vi "Charge_On_Magnet_Off.vi"() -> ()   [LabVIEW 2010]
uses:
  <vilib>/SwitchExecutive/nise.llb/niSE Multiconnect Mode Enum.ctl
  <instrlib>/Keithley 24XX/Keithley 24XX.lvlib
panel:
  in  "Apply Loads":bool
  out "Instruments Ready":bool
  in  "Release Instruments":bool
  in  "Initialize Instruments":bool
  in  "Apply Magnet":bool
  in  "Apply Charge":bool
  # "CHARGE"
  # "MAGNET"
  # "SETUP"
  # "LOADS"
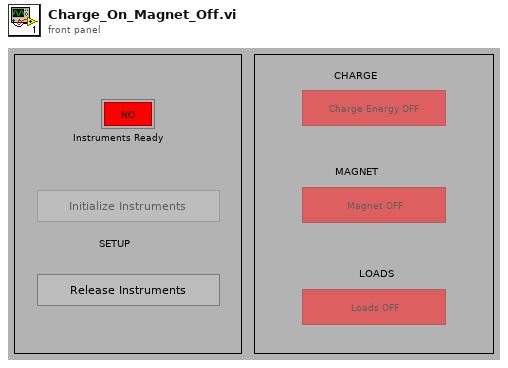
[diagram p1: front panel]
types:
  T1 = enum8{"Enabled", "Disabled", "Disabled and Grayed Out"}
  T2 = typedef "niSE Multiconnect Mode Enum.ctl" = i32
  T3 = typedef "niSE SessionRefnum.ctl" = refnum<k1>
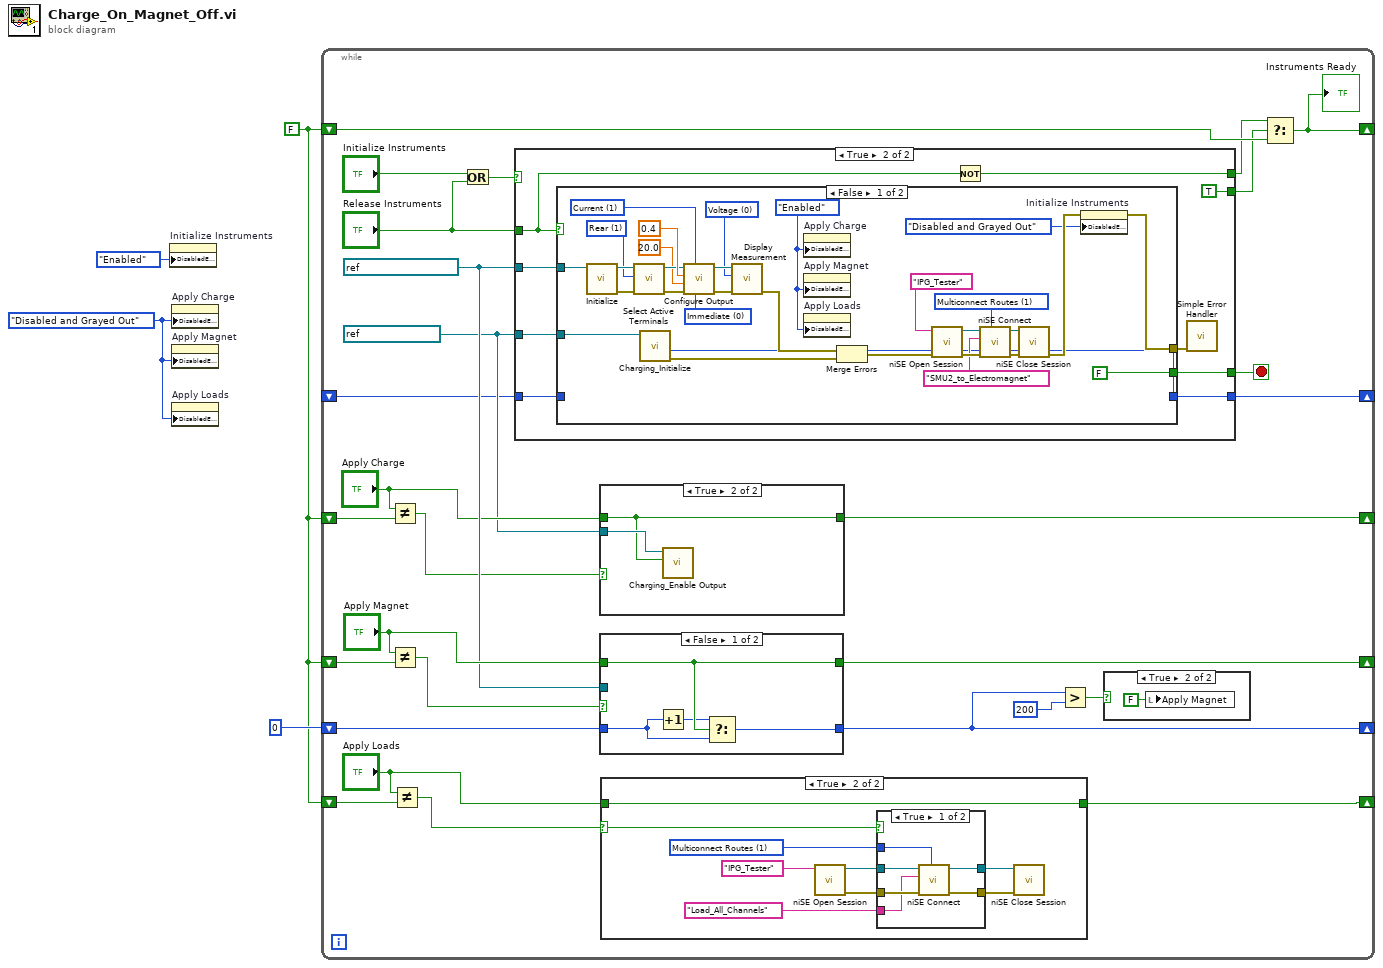
[diagram p0: block diagram]
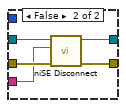
[diagram p3: hidden frame]
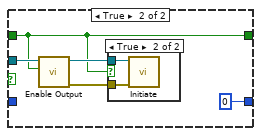
[diagram p6: hidden frame]
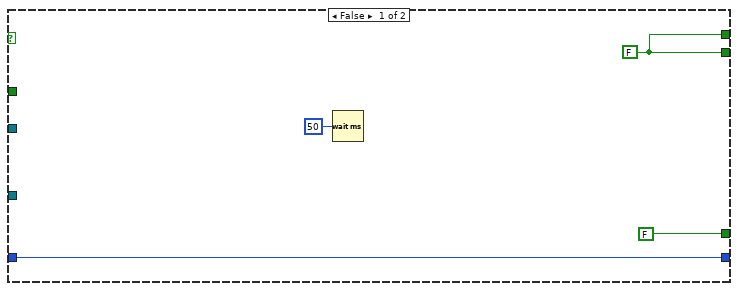
[diagram p8: hidden frame]
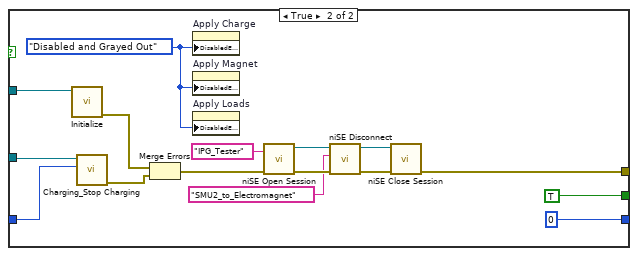
[diagram p9: hidden frame]
diagram:
  w1 = T1."Disabled and Grayed Out" ("Disabled")
  w2 = FALSE
  n1 = property on="Initialize Instruments" class="Bool"("DisabledEnum"=T1."Enabled" ("Disabled")) -> ()  [unwired: 2 in, 2 out]
  n2 = property on="Apply Charge" class="Bool (strict)"("DisabledEnum"=w1) -> ()  [unwired: 2 in, 2 out]
  n3 = property on="Apply Magnet" class="Bool (strict)"("DisabledEnum"=w1) -> ()  [unwired: 2 in, 2 out]
  n4 = property on="Apply Loads" class="Bool (strict)"("DisabledEnum"=w1) -> ()  [unwired: 2 in, 2 out]
  n5 = while {
    shift-right: [w32] -> _
    shift-left: w2 -> [w31]
    shift-right: [w13] -> _
    shift-left: w2 -> [w29]
    shift-right: [w19] -> _
    shift-left: w2 -> [w30]
    shift-right: [w17] -> _
    shift-left: u32 0 -> [w22]
    shift-right: [w8] -> _
    shift-left: w2 -> [w11]
    shift-right: [w6] -> _
    shift-left: _ -> [w5]
    stop <- w12 stop-if-true
    w7 = refnum<k15> "IVI-AG33210A" ("logical name (\"SampleFGen\")")
    w20 = refnum<visa-resource-name> "GPIB0::10::INSTR" ("VISA resource name")
    n6 = Not Equal?(x="Apply Charge", y=w29) -> (x != y?=w15:bool)
    n7 = Not Equal?(x="Apply Magnet", y=w30) -> (x != y?=w23:bool)
    n8 = Not Equal?(x="Apply Loads", y=w11) -> (x != y?=w10:bool)
    n9 = Or(x="Initialize Instruments", y="Release Instruments") -> (x .or. y?=w27:bool)
    n10 = case shown="True" w27 {
      tunnel: [w72 TRUE] -> w26
      tunnel: [w72 w80] -> w25
      tunnel: "Release Instruments" -> [_ w78]
      tunnel: w20 -> [_ w79]
      tunnel: w7 -> [_ w77]
      tunnel: [FALSE w75] -> w12
      tunnel: [w69 w74] -> w6
      tunnel: w5 -> [w69 w73]
      frame False {
        w72 = FALSE
        n11 = Wait (ms)(milliseconds to wait=u32 50) -> ()  [unwired: 1 out]
      }
      frame True {
        n12 = case shown="False" w78 {
          tunnel: w79 -> [w111 w127]
          tunnel: w77 -> [w82 w115]
          tunnel: [w87 w120] -> w76
          tunnel: [FALSE TRUE] -> w75
          tunnel: [w83 0 ("Arbitrary Waveform Handle [ARB]")] -> w74
          tunnel: w73 -> [_ w112]
          frame False {
            w91 = u16 0 items=["Immediate", "Triggered"] ("Output Type  (0: Immediate)")
            w92 = u16 0 items=["Voltage", "Current", "Resistance"] ("Displayed Measurement (0: Voltage)")
            w85 = T1."Enabled" ("Disabled")
            w101 = T2 1 items=["Use Default Mode"=-1, "Multiconnect Routes"=1, "No Multiconnect"=0] ("Multiconnect Mode (Use Default Mode)")
            w103 = u16 1 items=["Voltage", "Current"] ("Source Mode  (0: Voltage)")
            w108 = u16 1 items=["Front", "Rear"] ("Active Terminals (0: Front)")
            n13 = call <instrlib>:"Initialize.vi"("VISA resource name"=w111) -> ("error out"=w110:errorcluster, "VISA resource name out"=w109:refnum<visa-resource-name>)  [unwired: 9 in]
            n14 = call <instrlib>:"Select Active Terminals.vi"("error in (no error)"=w110, "Active Terminals (0: Front)"=w108, "VISA resource name"=w109) -> ("error out"=w105:errorcluster, "VISA resource name out"=w106:refnum<visa-resource-name>)  [unwired: 7 in]
            n15 = call "Charging_Initialize.vi"("logical name (\"SampleFGen\")"=w82) -> ("error out"=w84:errorcluster, "Arbitrary Waveform Handle [ARB]"=w83:i32)  [unwired: 8 in, 1 out]
            n16 = call <instrlib>:"Configure Output.vi"("Output Type  (0: Immediate)"=w91, "Source Mode  (0: Voltage)"=w103, "error in (no error)"=w105, "Compliance  Level (0.1)"=20.0, "Output Level (0)"=0.4, "VISA resource name"=w106) -> ("error out"=w94:errorcluster, "VISA resource name out"=w93:refnum<visa-resource-name>)  [unwired: 4 in]
            n17 = call <instrlib>:"Display Measurement.vi"("error in (no error)"=w94, "Displayed Measurement (0: Voltage)"=w92, "VISA resource name"=w93) -> ("error out"=w90:errorcluster)  [unwired: 7 in, 1 out]
            n18 = property on="Apply Charge" class="Bool (strict)"("DisabledEnum"=w85) -> ()  [unwired: 2 in, 2 out]
            n19 = property on="Apply Magnet" class="Bool (strict)"("DisabledEnum"=w85) -> ()  [unwired: 2 in, 2 out]
            n20 = property on="Apply Loads" class="Bool (strict)"("DisabledEnum"=w85) -> ()  [unwired: 2 in, 2 out]
            n21 = Merge Errors(w90, w84) -> (w95:errorcluster)
            n22 = call <vilib>:"niSE Open Session.vi"("error in (no error)"=w95, "Virtual Device Name (SwitchConfiguration1)"="IPG_Tester") -> ("error out"=w99:errorcluster, "NISE Session (out)"=w102:T3)  [unwired: 4 in]
            n23 = call <vilib>:"niSE Connect.vi"("Multiconnect Mode (Use Default Mode)"=w101, "error in (no error)"=w99, "Connection Specification (\"\")"="SMU2_to_Electromagnet" ("Connection Specification (\"\")"), "NISE Session (in)"=w102) -> ("error out"=w96:errorcluster, "NISE Session (out)"=w97:T3)  [unwired: 6 in]
            n24 = call <vilib>:"niSE Close Session.vi"("error in (no error)"=w96, "NISE Session (in)"=w97) -> ("error out"=w88:errorcluster)  [unwired: 5 in]
            n25 = property on="Initialize Instruments" class="Bool"(error in=w88, "DisabledEnum"=T1."Disabled and Grayed Out" ("Disabled")) -> (error out=w87:errorcluster)  [unwired: 1 in, 1 out]
          }
          frame True {
            w116 = T1."Disabled and Grayed Out" ("Disabled")
            n26 = call <instrlib>:"Initialize.vi"("VISA resource name"=w127) -> ("error out"=w121:errorcluster)  [unwired: 9 in, 1 out]
            n27 = call "Charging_Stop Charging.vi"("waveform handle (0)"=w112, "logical name (\"SampleFGen\")"=w115) -> ("error out"=w114:errorcluster)  [unwired: 9 in]
            n28 = Merge Errors(w121, w114) -> (w122:errorcluster)
            n29 = property on="Apply Charge" class="Bool (strict)"("DisabledEnum"=w116) -> ()  [unwired: 2 in, 2 out]
            n30 = property on="Apply Magnet" class="Bool (strict)"("DisabledEnum"=w116) -> ()  [unwired: 2 in, 2 out]
            n31 = property on="Apply Loads" class="Bool (strict)"("DisabledEnum"=w116) -> ()  [unwired: 2 in, 2 out]
            n32 = call <vilib>:"niSE Open Session.vi"("error in (no error)"=w122, "Virtual Device Name (SwitchConfiguration1)"="IPG_Tester") -> ("error out"=w124:errorcluster, "NISE Session (out)"=w126:T3)  [unwired: 4 in]
            n33 = call <vilib>:"niSE Disconnect.vi"("error in (no error)"=w124, "Disconnection Specification (\"\")"="SMU2_to_Electromagnet" ("Connection Specification (\"\")"), "NISE Session (in)"=w126) -> ("error out"=w117:errorcluster, "NISE Session (out)"=w123:T3)  [unwired: 3 in]
            n34 = call <vilib>:"niSE Close Session.vi"("error in (no error)"=w117, "NISE Session (in)"=w123) -> ("error out"=w120:errorcluster)  [unwired: 5 in]
          }
        }
        n35 = Not(x=w78) -> (.not. x?=w80:bool)
        n36 = call <vilib>:"Simple Error Handler.vi"("error in (no error)"=w76) -> ()  [unwired: 4 in, 5 out]
      }
    }
    n37 = case shown="True" w15 {
      tunnel: w7 -> [_ w56]
      tunnel: "Apply Charge" -> [w54 w55]
      tunnel: [w54 w55] -> w13
      frame False {
      }
      frame True {
        n38 = call "Charging_Enable Output.vi"("enable output (true)"=w55, "instrument handle"=w56) -> ()  [unwired: 8 in, 2 out]
      }
    }
    n39 = case shown="False" w23 {
      tunnel: w22 -> [w58 _]
      tunnel: [w61 u32 0] -> w17
      tunnel: "Apply Magnet" -> [w60 w62]
      tunnel: w20 -> [_ w66]
      tunnel: [w60 w62] -> w19
      frame False {
        n40 = Increment(x=w58) -> (x+1=w59:u32)
        n41 = Select(t=w59, s=w60, f=w58) -> (s? t:f=w61:u32)
      }
      frame True {
        n42 = call <instrlib>:"Enable Output.vi"("Enable Output (T: Enable)"=w62, "VISA resource name"=w66) -> ("error out"=w64:errorcluster, "VISA resource name out"=w63:refnum<visa-resource-name>)  [unwired: 8 in]
        n43 = case shown="True" w62 {
          tunnel: w64 -> [_ w68]
          tunnel: w63 -> [_ w67]
          frame False {
          }
          frame True {
            n44 = call <instrlib>:"Initiate.vi"("error in (no error)"=w68, "VISA resource name"=w67) -> ()  [unwired: 8 in, 2 out]
          }
        }
      }
    }
    n45 = case shown="True" w10 {
      selector: w10 -> [_ w34]
      tunnel: "Apply Loads" -> [w33 w42]
      tunnel: [w33 w42] -> w8
      frame False {
      }
      frame True {
        w40 = T2 1 items=["Use Default Mode"=-1, "Multiconnect Routes"=1, "No Multiconnect"=0] ("Multiconnect Mode (Use Default Mode)")
        n46 = call <vilib>:"niSE Open Session.vi"("Virtual Device Name (SwitchConfiguration1)"="IPG_Tester") -> ("error out"=w39:errorcluster, "NISE Session (out)"=w41:T3)  [unwired: 5 in]
        n47 = case shown="True" w34 {
          tunnel: w41 -> [w48 w53]
          tunnel: w40 -> [w47 _]
          tunnel: w39 -> [w46 w52]
          tunnel: "Load_All_Channels" ("Connection Specification (\"\")") -> [w45 w51]
          tunnel: [w44 w50] -> w37
          tunnel: [w43 w49] -> w36
          frame True {
            n48 = call <vilib>:"niSE Connect.vi"("Multiconnect Mode (Use Default Mode)"=w47, "error in (no error)"=w46, "Connection Specification (\"\")"=w45, "NISE Session (in)"=w48) -> ("error out"=w43:errorcluster, "NISE Session (out)"=w44:T3)  [unwired: 6 in]
          }
          frame False {
            n49 = call <vilib>:"niSE Disconnect.vi"("error in (no error)"=w52, "Disconnection Specification (\"\")"=w51, "NISE Session (in)"=w53) -> ("error out"=w49:errorcluster, "NISE Session (out)"=w50:T3)  [unwired: 3 in]
          }
        }
        n50 = call <vilib>:"niSE Close Session.vi"("error in (no error)"=w36, "NISE Session (in)"=w37) -> ()  [unwired: 5 in, 1 out]
      }
    }
    n51 = Greater?(x=w17, y=u32 200) -> (0:w18:bool)
    n52 = case shown="True" w18 {
      frame False {
      }
      frame True {
        n53 = local write "Apply Magnet"(FALSE) -> ()
      }
    }
    n54 = Select(t=w25, s=w26, f=w31) -> (s? t:f=w32:bool)
    "Instruments Ready" <- w32
  }
